vi "Add_length_to_string.vi"(1 "String in":string) -> (0 "String out":string)   [LabVIEW 2016]
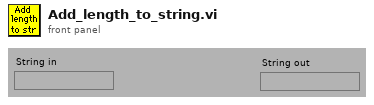
[diagram p1: front panel]
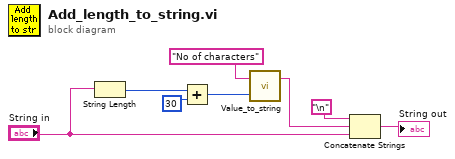
[diagram p0: block diagram]
diagram:
  n1 = String Length(string="String in") -> (length=w4:i32)
  n2 = Add(x=w4, y=30) -> (x+y=w2:i32)
  n3 = call "Value_to_string.vi"("Value"=w2, "Label for value"="No of characters" ("Variable name")) -> ("Output string"=w7:string)  [unwired: 1 in]
  n4 = Concatenate Strings("\n", w7, "String in") -> (→"String out":string)
